vi "RP ADC to Volts 2D.vi"(6 "osc_fpga_cnv_cnt_to_v method":bool, 7 "Max Volts":sgl=1.0, 11 "ADC data":i16[][](array[numeric])) -> (3 "Volts":sgl[][](array[numeric]))   [LabVIEW 2015]
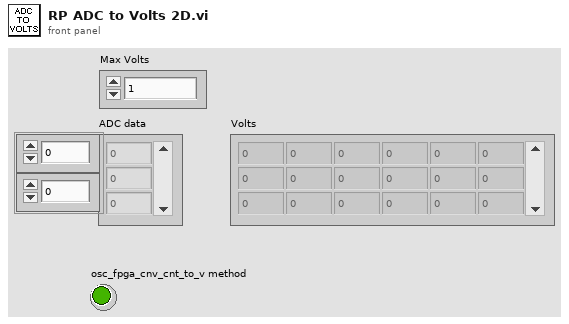
[diagram p1: front panel]
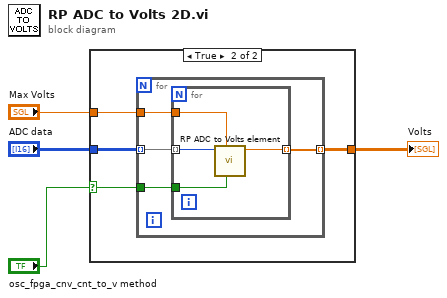
[diagram p0: block diagram]
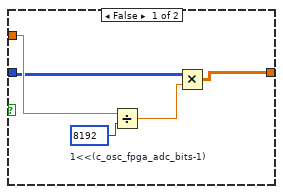
[diagram p2: hidden frame]
diagram:
  n1 = case shown="True" "osc_fpga_cnv_cnt_to_v method" {
    selector: "osc_fpga_cnv_cnt_to_v method" -> [_ w10]
    tunnel: "ADC data" -> [w6 w13]
    tunnel: [w5 w12] -> w3
    tunnel: "Max Volts" -> [w8 w11]
    frame False {
      w9 = 8192  # 1<<(c_osc_fpga_adc_bits-1)
      n2 = Divide(x=w8, y=w9) -> (x/y=w7:sgl)
      n3 = Multiply(x=w6, y=w7) -> (x*y=w5:sgl[][])
    }
    frame True {
      n4 = for {
        tunnel: w13 -> [w17] mode=indexing
        tunnel: [w16] -> w12 mode=indexing
        tunnel: w10 -> [w15]
        tunnel: w11 -> [w14]
        n5 = for {
          tunnel: w17 -> [w21] mode=indexing
          tunnel: [w20] -> w16 mode=indexing
          tunnel: w15 -> [w19]
          tunnel: w14 -> [w18]
          n6 = call "RP ADC to Volts element.vi"("osc_fpga_cnv_cnt_to_v method"=w19, "Max Volts"=w18, "ADC data"=w21) -> ("Volts"=w20:sgl)  [unwired: 8 in]
        }
      }
    }
  }
  "Volts" <- w3
